vi "Save IoT Configuration to DB.vi"(7 "error in":errorcluster, 9 "IoT Configuration cluster":T1, 10 "GTron DB":path=path "D:/SQL Database/Gtron Database.db") -> (0 "error out":errorcluster)   [LabVIEW 2019, in "DataLogger.lvclass"]
uses:
  DataLogger.lvclass
  <vilib>/drjdpowell/SQLite Library/SQL Statement/SQL Statement.lvclass
  <vilib>/drjdpowell/SQLite Library/SQL Connection/Connection.lvclass
  <vilib>/drjdpowell/SQLite Library/SQL Connection/Open (path).vi
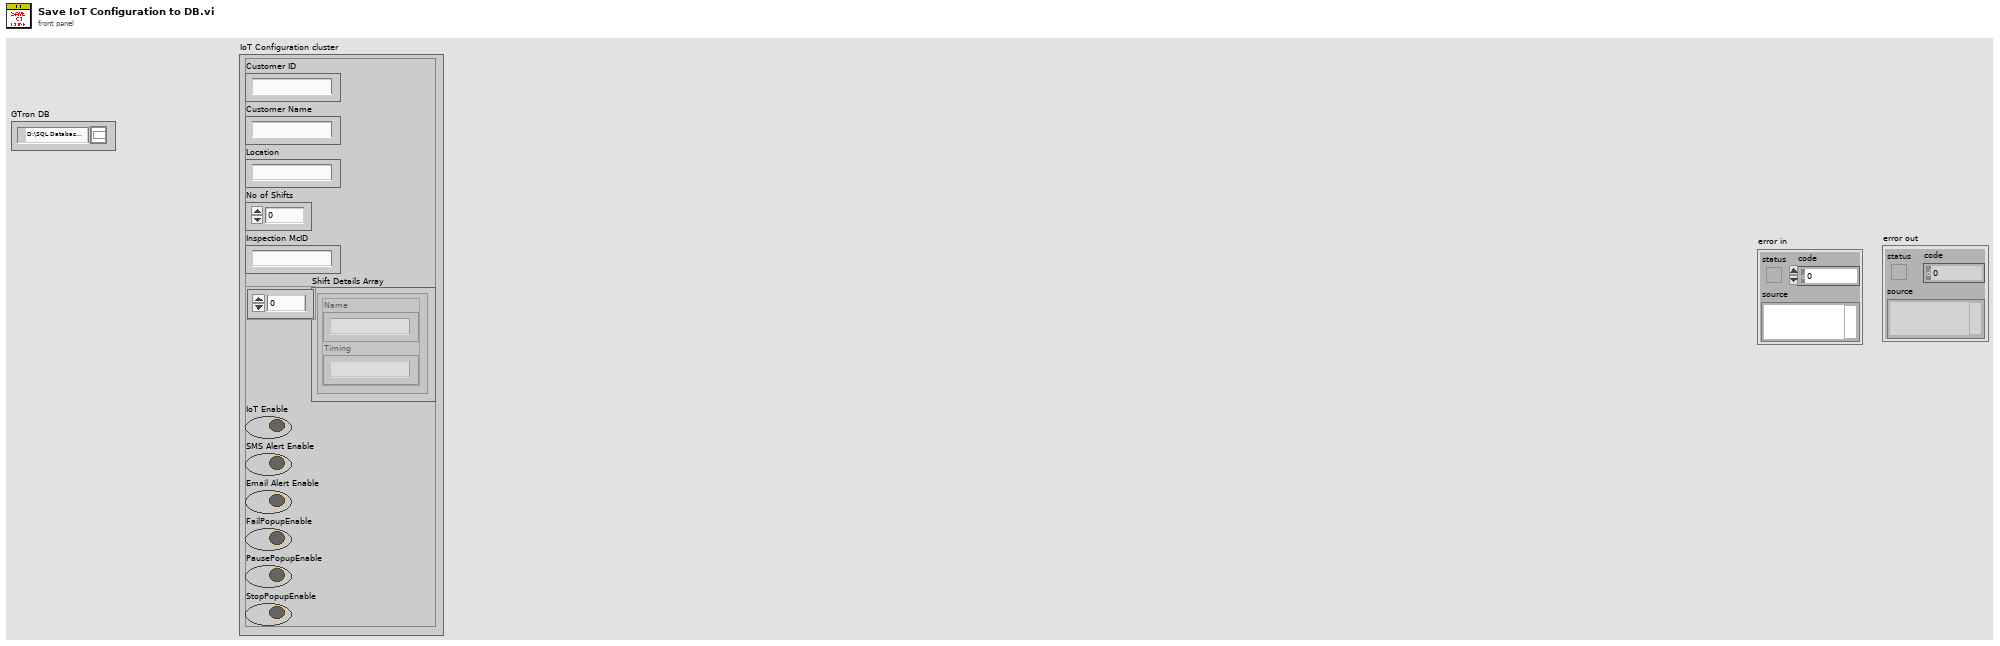
[diagram p1: front panel]
types:
  T1 = cluster{"Customer ID":string, "Customer Name":string, "Location":string, "No of Shifts":u8, "Inspection McID":string, "Shift Details Array":cluster{"Name":string, "Timing":string}[], "IoT Enable":bool, "SMS Alert Enable":bool, "Email Alert Enable":bool, "FailPopupEnable":bool, "PausePopupEnable":bool, "StopPopupEnable":bool}
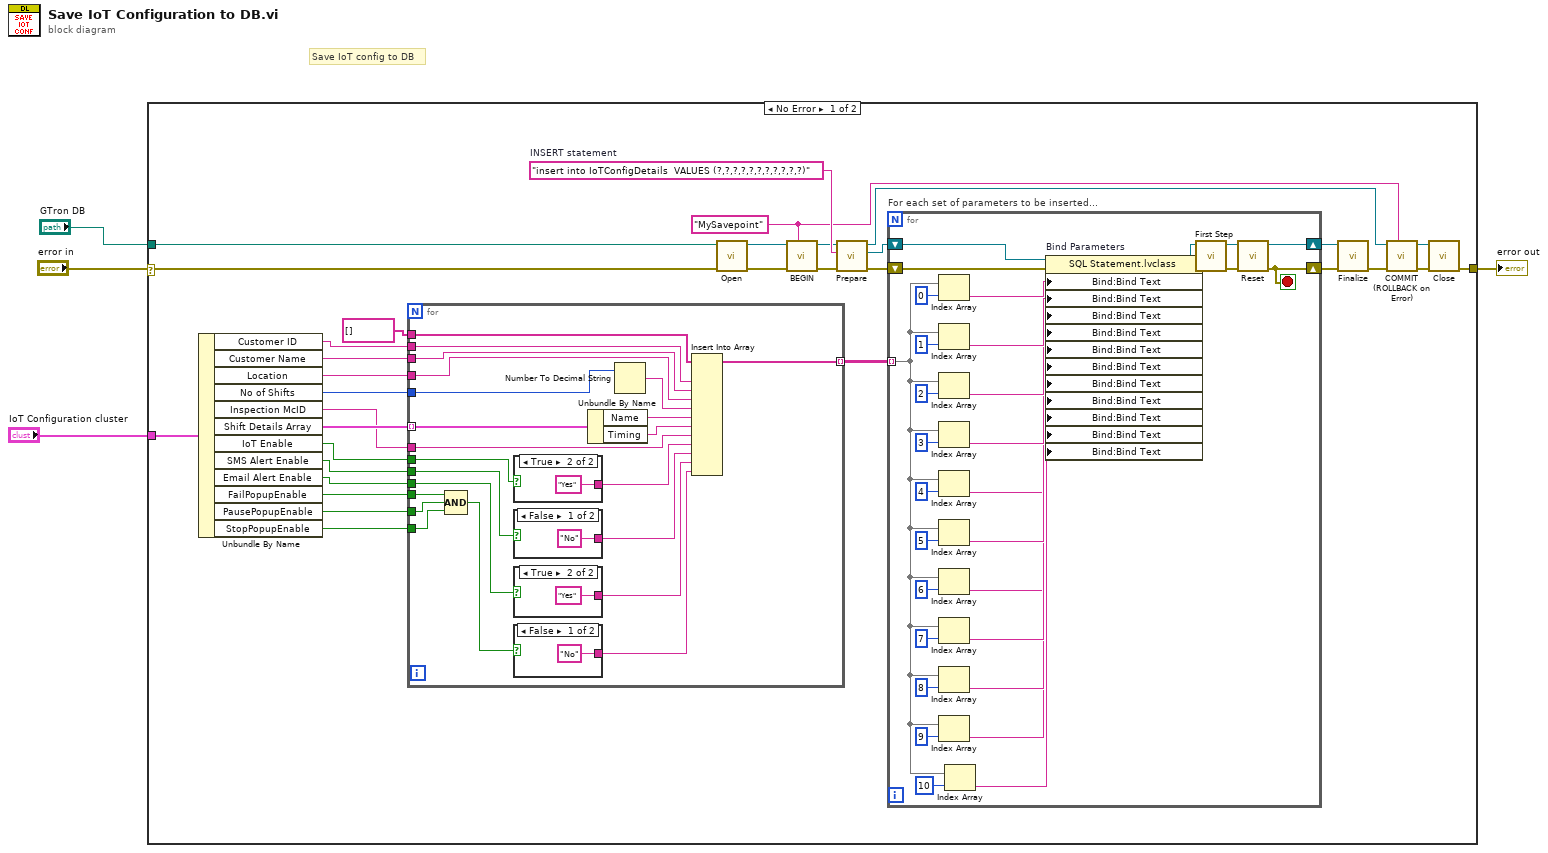
[diagram p0: block diagram]
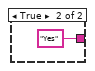
[diagram p2: hidden frame]
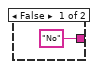
[diagram p3: hidden frame]
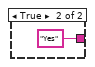
[diagram p4: hidden frame]
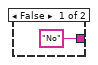
[diagram p5: hidden frame]
diagram:
  # "Save IoT config to DB"
  n1 = case shown="No Error" "error in" {
    selector: "error in" -> [w5 w98]
    tunnel: [w12 w98] -> w4
    tunnel: "GTron DB" -> [w11 _]
    tunnel: "IoT Configuration cluster" -> [w8 _]
    frame No Error {
      w17 = "MySavepoint" ("Savepoint name")
      w22 = "insert into IoTConfigDetails  VALUES (?,?,?,?,?,?,?,?,?,?,?)"  # INSERT statement
      n2 = Unbundle By Name(w8) -> ("Customer ID"=w35:string, "Customer Name"=w34:string, "Location"=w33:string, "No of Shifts"=w32:u8, "Inspection McID"=w31:string, "Shift Details Array"=w36:cluster{"Name":string, "Timing":string}[], "IoT Enable"=w30:bool, "SMS Alert Enable"=w29:bool, "Email Alert Enable"=w28:bool, "FailPopupEnable"=w9:bool, "PausePopupEnable"=w7:bool, "StopPopupEnable"=w6:bool)
      n3 = for {
        tunnel: w36 -> [w84] mode=indexing
        tunnel: w35 -> [w89]
        tunnel: w34 -> [w88]
        tunnel: w33 -> [w87]
        tunnel: w32 -> [w86]
        tunnel: w31 -> [w72]
        tunnel: w30 -> [w83]
        tunnel: w29 -> [w81]
        tunnel: w28 -> [w80]
        tunnel: [w77] -> w10 mode=indexing
        tunnel: string[] [] -> [w76]
        tunnel: w9 -> [w71]
        tunnel: w7 -> [w69]
        tunnel: w6 -> [w70]
        n4 = Compound Arithmetic op=AND(w71, w69, w70) -> (w68:bool)
        n5 = case shown="True" w83 {
          tunnel: ["No" "Yes"] -> w82
          frame False {
          }
          frame True {
          }
        }
        n6 = case shown="False" w81 {
          tunnel: ["No" "Yes"] -> w79
          frame False {
          }
          frame True {
          }
        }
        n7 = case shown="True" w80 {
          tunnel: ["No" "Yes"] -> w78
          frame False {
          }
          frame True {
          }
        }
        n8 = case shown="False" w68 {
          tunnel: ["No" "Yes"] -> w75
          frame False {
          }
          frame True {
          }
        }
        n9 = Unbundle By Name(w84) -> ("Name"=w74:string, "Timing"=w73:string)
        n10 = Number To Decimal String(number=w86) -> (decimal integer string=w85:string)  [unwired: 1 in]
        n11 = Insert Into Array "Insert Into Array"(array=w76, new element #1=w89, new element #2=w88, new element #3=w87, new element #4=w85, new element #5=w74, new element #6=w73, new element #7=w72, new element #8=w82, new element #9=w79, new element #10=w78, new element #11=w75) -> (w77:string[])  [unwired: 1 in]
      }
      n12 = call-poly <vilib>:"Open.vi"("error in (no error)"=w5, "db file"=w11) -> ("error out"=w26:errorcluster, "SQLite Connection"=w25:refnum<class "Connection.lvclass">)  [unwired: 8 in]
      n13 = call <vilib>:"BEGIN.vi"("Savepoint name"=w17, "error in (no error)"=w26, "Connection in"=w25) -> ("error out"=w18:errorcluster, "Connection out"=w19:refnum<class "Connection.lvclass">)  [unwired: 7 in]
      n14 = call <vilib>:"Prepare.vi"("error in (no error)"=w18, "SQL"=w22, "SQLite Connection in"=w19) -> ("error out"=w23:errorcluster, "SQL Statement"=w24:refnum<class "SQL Statement.lvclass">, "SQLite Connection"=w16:refnum<class "Connection.lvclass">)  [unwired: 4 in, 2 out]
      n15 = for "For each set of parameters to be inserted..." {
        shift-right: [w65] -> w21
        shift-left: w24 -> [w67]
        shift-right: [w64] -> w20
        shift-left: w23 -> [w66]
        tunnel: w10 -> [w39] mode=indexing
        stop <- w64 stop-if-true
        n16 = Index Array(array=w39, index=0) -> (element=w52:string)
        n17 = Index Array(array=w39, index=1) -> (element=w51:string)
        n18 = Index Array(array=w39, index=2) -> (element=w50:string)
        n19 = Index Array(array=w39, index=3) -> (element=w49:string)
        n20 = Index Array(array=w39, index=4) -> (element=w38:string)
        n21 = Index Array(array=w39, index=5) -> (element=w48:string)
        n22 = Index Array(array=w39, index=6) -> (element=w37:string)
        n23 = Index Array(array=w39, index=7) -> (element=w44:string)
        n24 = Index Array(array=w39, index=8) -> (element=w43:string)
        n25 = Index Array(array=w39, index=9) -> (element=w42:string)
        n26 = Index Array(array=w39, index=10) -> (element=w40:string)
        n27 = property on="Bind Parameters" class="SQL Statement.lvclass"(reference=w67, error in=w66, "Bind:Bind Text"=w52, "Bind:Bind Text"=w51, "Bind:Bind Text"=w50, "Bind:Bind Text"=w49, "Bind:Bind Text"=w38, "Bind:Bind Text"=w48, "Bind:Bind Text"=w37, "Bind:Bind Text"=w44, "Bind:Bind Text"=w43, "Bind:Bind Text"=w42, "Bind:Bind Text"=w40) -> (reference out=w63:refnum<class "SQL Statement.lvclass">, error out=w62:errorcluster)
        n28 = call <vilib>:"First Step.vi"("error in (no error)"=w62, "SQL Statement in"=w63) -> ("error out"=w61:errorcluster, "SQL Statement"=w60:refnum<class "SQL Statement.lvclass">)  [unwired: 7 in, 1 out]
        n29 = call <vilib>:"Reset.vi"("error in (no error)"=w61, "SQL Statement in"=w60) -> ("error out"=w64:errorcluster, "SQL Statement"=w65:refnum<class "SQL Statement.lvclass">)  [unwired: 8 in]
      }
      n30 = call <vilib>:"Finalize.vi"("error in (no error)"=w20, "SQL Statement in"=w21) -> ("error out"=w15:errorcluster)  [unwired: 9 in]
      n31 = call <vilib>:"COMMIT (ROLLBACK on Error).vi"("Savepoint name"=w17, "error in (no error)"=w15, "Connection in"=w16) -> ("error out"=w14:errorcluster, "Connection out"=w13:refnum<class "Connection.lvclass">)  [unwired: 7 in]
      n32 = call-dynamic "Close.vi"("error in (no error)"=w14, "SQLite Connection in"=w13) -> ("error out"=w12:errorcluster)  [unwired: 9 in]
    }
    frame Error {
    }
  }
  "error out" <- w4
